vi "ADIS16470 Scale Data.vi"(3 "TimeStamp":u32, 5 "Data In":u8[](array[numeric])) -> (1 "Scaled Data Out":dbl[](array[numeric]))   [LabVIEW 2019]
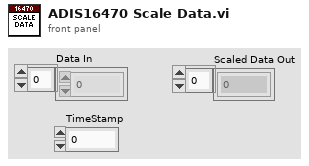
[diagram p1: front panel]
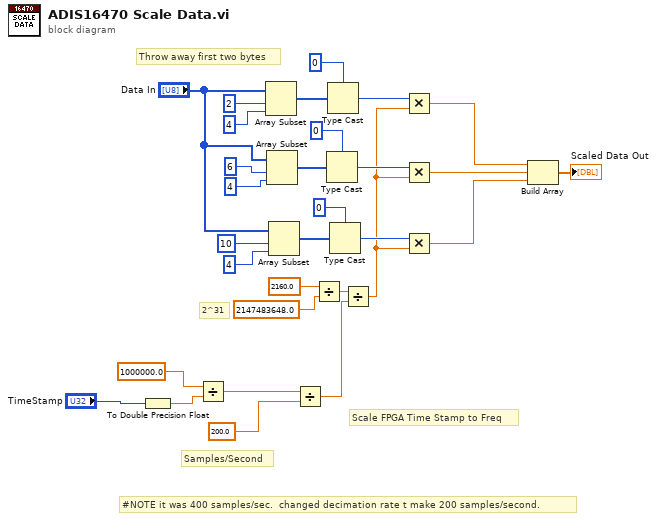
[diagram p0: block diagram]
diagram:
  # "Samples/Second"
  # "#NOTE it was 400 samples/sec.  changed decimation rate t make 200 samples/second."
  # "Scale FPGA Time Stamp to Freq"
  # "2^31"
  # "Throw away first two bytes"
  n1 = To Double Precision Float(number="TimeStamp") -> (double precision float=w5:dbl)
  n2 = Divide(x=1000000.0, y=w5) -> (x/y=w7:dbl)
  n3 = Array Subset(array="Data In", index=2, length=4) -> (w23:u8[])
  n4 = Array Subset(array="Data In", index=6, length=4 ("index")) -> (w21:u8[])
  n5 = Array Subset(array="Data In", index=10, length=4) -> (w22:u8[])
  n6 = Divide(x=w7, y=200.0) -> (x/y=w8:dbl)
  n7 = Divide(x=2160.0, y=2147483648.0) -> (x/y=w10:dbl)
  n8 = Type Cast(type=0, x=w21) -> (*(type *) &x=w15:i32)
  n9 = Type Cast(type=0, x=w23) -> (*(type *) &x=w17:i32)
  n10 = Type Cast(type=0, x=w22) -> (*(type *) &x=w16:i32)
  n11 = Divide(x=w10, y=w8) -> (x/y=w9:dbl)
  n12 = Multiply(x=w17, y=w9) -> (x*y=w3:dbl)
  n13 = Multiply(x=w15, y=w9) -> (x*y=w2:dbl)
  n14 = Multiply(x=w16, y=w9) -> (x*y=w1:dbl)
  n15 = Build Array(w3, w2, w1) -> (→"Scaled Data Out":dbl[])
